vi "LittleBoatHindbrainAct.vi"(10 "NotifierReff":T1, 11 "VISA Refnum in":refnum<visa-resource-name>) -> (0 "error out":errorcluster)   [LabVIEW 2013]
uses:
  Data/TypeDefs/Notifiers.ctl
  Data/TypeDefs/UTM Location.ctl
  Data/TypeDefs/Sail Set Suggestions.ctl
  Data/TypeDefs/Rudder Set Suggestions.ctl
  Data/TypeDefs/OverrideInformation.ctl
  Data/TypeDefs/OverrideMode.ctl
  Data/TypeDefs/MotorSetup.ctl
  Data/TypeDefs/DynamixelSetupInfo.ctl
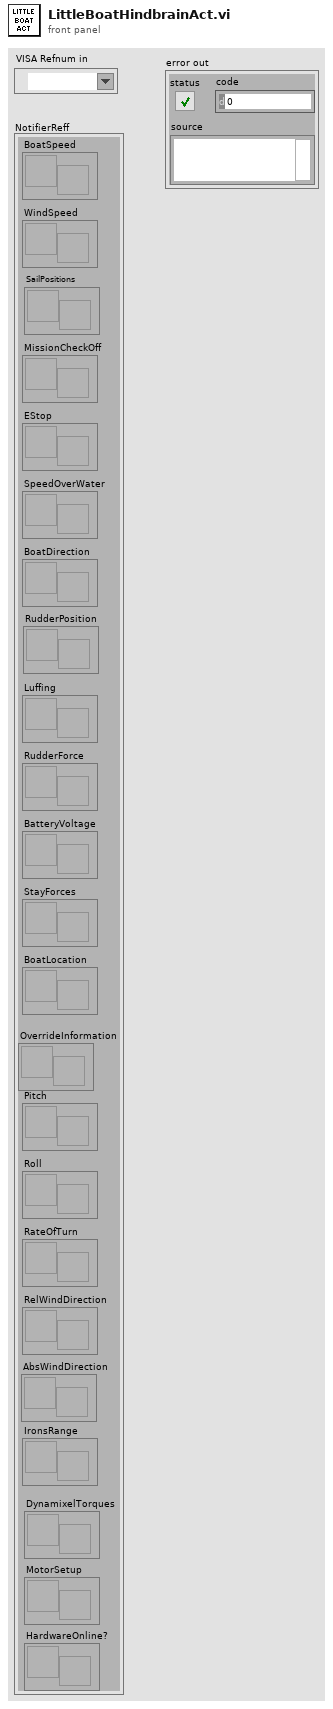
[diagram p1: front panel]
types:
  T1 = typedef "Notifiers.ctl" = cluster{"BoatSpeed":refnum<notifier>, "WindSpeed":refnum<notifier>, "MissionCheckOff":refnum<notifier>, "EStop":refnum<notifier>, "SpeedOverWater":refnum<notifier>, "BoatDirection":refnum<notifier>, "Luffing":refnum<notifier>, "RudderForce":refnum<notifier>, "BatteryVoltage":refnum<notifier>, "StayForces":refnum<notifier>, "BoatLocation":refnum<notifier>, "Pitch":refnum<notifier>, "Roll":refnum<notifier>, "RateOfTurn":refnum<notifier>, "RelWindDirection":refnum<notifier>, "SailPositions":refnum<notifier>, "RudderPosition":refnum<notifier>, "IronsRange":refnum<notifier>, "AbsWindDirection":refnum<notifier>, "OverrideInformation":refnum<notifier>, "DynamixelTorques":refnum<notifier>, "MotorSetup":refnum<notifier>, "HardwareOnline?":refnum<notifier>}
  T2 = typedef "Sail Set Suggestions.ctl" = cluster{"MainSailSuggestion":dbl, "JibSailSuggestion":dbl}
  T3 = typedef "Rudder Set Suggestions.ctl" = dbl
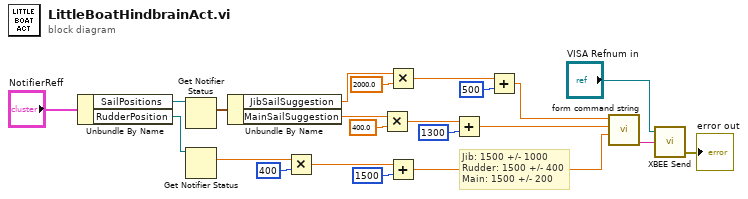
[diagram p0: block diagram]
diagram:
  # "Jib: 1500 +/- 1000\nRudder: 1500 +/- 400\nMain: 1500 +/- 200"
  n1 = Unbundle By Name("NotifierReff") -> ("SailPositions"=w4:refnum<notifier>, "RudderPosition"=w5:refnum<notifier>)
  n2 = Get Notifier Status(notifier=w4) -> (current notification=w7:T2)  [unwired: 1 in, 4 out]
  n3 = Get Notifier Status(notifier=w5) -> (current notification=w9:T3)  [unwired: 1 in, 4 out]
  n4 = Unbundle By Name(w7) -> ("JibSailSuggestion"=w15:dbl, "MainSailSuggestion"=w22:dbl)
  n5 = Multiply(x=w9, y=400) -> (x*y=w11:T3)
  n6 = Multiply(x=w22, y=400.0) -> (x*y=w20:dbl)
  n7 = Multiply(x=w15, y=2000.0) -> (x*y=w16:dbl)
  n8 = Add(x=w11, y=1500) -> (x+y=w12:T3)
  n9 = Add(x=w20, y=1300) -> (x+y=w21:dbl)
  n10 = Add(x=w16, y=500) -> (x+y=w17:dbl)
  n11 = call "form command string.vi"("Rudder"=w12, "Main sheet"=w21, "Jib Sheet"=w17) -> ("String"=w1:string)  [unwired: 5 in, 3 out]
  n12 = call "XBEE Send.vi"("String"=w1, "VISA resource name"="VISA Refnum in") -> ("error out"=→"error out":errorcluster)  [unwired: 1 in, 2 out]
